vi "S7COMM - Response Error Code-error.vi"() -> (0 "error out":errorcluster)   [LabVIEW 2014, in "S7NetCom.lvclass"]
uses:
  S7NetCom.lvclass
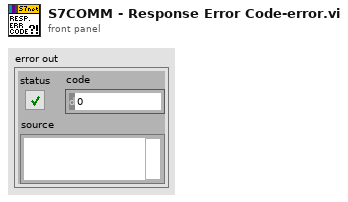
[diagram p1: front panel]
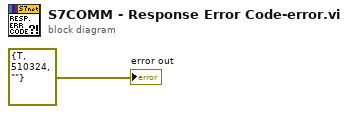
[diagram p0: block diagram]
diagram:
  "error out" <- errorcluster {"status"=TRUE, "code"=510324, "source"=""} ("error IO")
